vi "Config.vi"(8 "error in (no error)":errorcluster, 10 "Setting":T1={"Resolution (Digits)"=5.5, "Current Source (Amps)"=0.001, "Range"=2.0, "Measurement Type"=enum."DC Volts"} {"Range" format="%.2p"; "Current Source (Amps)" items=["1uA"=1e-06, "10uA"=1e-05, "100uA"=0.0001, "1mA"=0.001]; "Resolution (Digits)" items=["3 1/2"=3.5, "4 1/2"=4.5, "5 1/2"=5.5, "6 1/2"=6.5, "7 1/2"=7.5]}, 11 "DMM in":refnum<class "MIO.lvclass">) -> (0 "error out":errorcluster, 3 "DMM out":refnum<class "MIO.lvclass">)   [LabVIEW 2019, in "Hardware Abstration.lvlib" / "MIO.lvclass"]
uses:
  MIO.lvclass
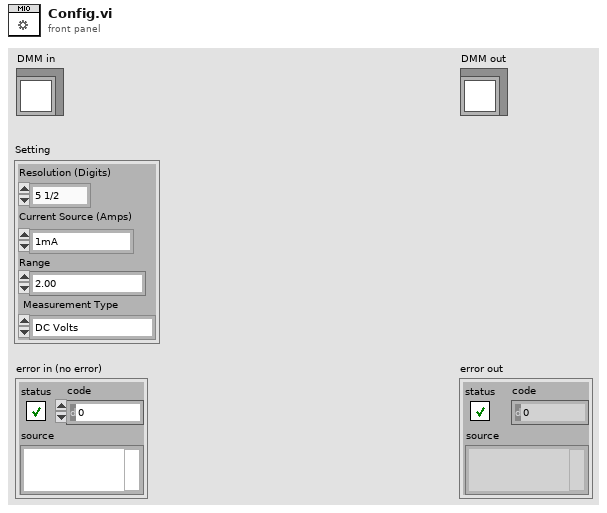
[diagram p1: front panel]
types:
  T1 = cluster{"Resolution (Digits)":dbl, "Current Source (Amps)":dbl, "Range":dbl, "Measurement Type":enum16{"DC Volts", "AC Volts", "DC Current", "AC Current", "2-wire Resistance", "4-wire Resistance", "Diode", "Frequency", "Period", "AC Volts DC Coupled", "Capacitance", "Inductance", "Temperature"}}
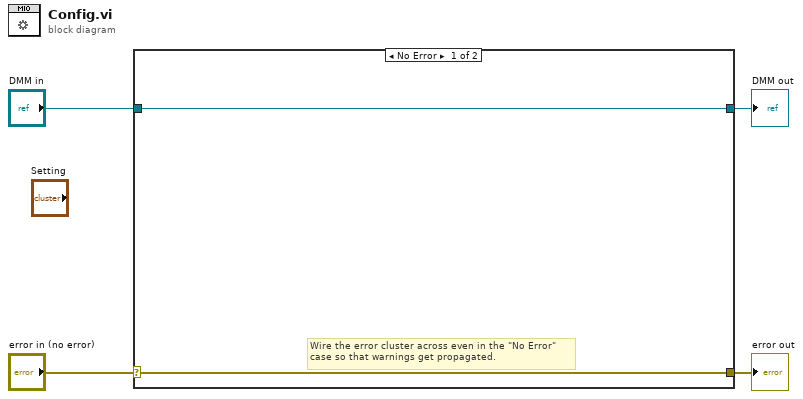
[diagram p0: block diagram]
diagram:
  n1 = case shown="No Error" "error in (no error)" {
    selector: "error in (no error)" -> [w5 w8]
    tunnel: [w5 w8] -> w3
    tunnel: [w6 w7] -> w1
    tunnel: "DMM in" -> [w6 w7]
    frame No Error {
      # "Wire the error cluster across even in the \"No Error\"\ncase so that warnings get propagated."
    }
    frame Error {
    }
  }
  "error out" <- w3
  "DMM out" <- w1
